vi "BlueToothOn.vi"(0 "NXT/EV3":T1, 1 "Connection":u8, 2 "Partner Name":string) -> (3 "NXT/EV3 2":T1, 4 "Connection":u8=1, 5 "Partner Name":string="Client", 6 "Success":bool)   [LabVIEW 2013]
uses:
  <vilib>/NXT/Subs/LVHSConnector.ctl
  <vilib>/NXT/LegoClasses/BrickReference/BrickReference.lvclass
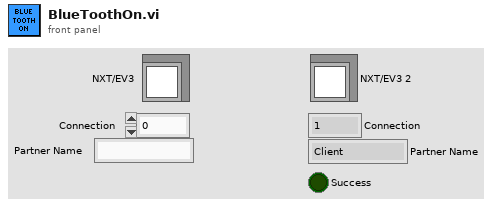
[diagram p1: front panel]
types:
  T1 = typedef "LVHSConnector.ctl" = refnum<class "BrickReference.lvclass">
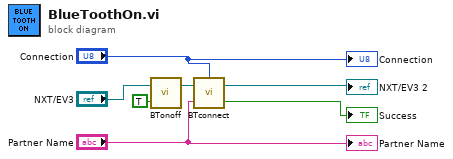
[diagram p0: block diagram]
diagram:
  n1 = call <vilib>:"BTonoff.vi"("On/Off"=TRUE, "NXT/EV3"="NXT/EV3") -> ("NXT/EV3"=w7:T1)  [unwired: 1 in, 1 out]
  n2 = call <vilib>:"BTconnect.vi"("Partner Name"="Partner Name", "NXT/EV3"=w7, "Connection"="Connection") -> ("Success"=→"Success":bool, "NXT/EV3"=→"NXT/EV3 2":T1)
  "Connection" <- "Connection"
  "Partner Name" <- "Partner Name"
